vi "VCS Add Pvt Value To Ipm Buffer.vi"(0 "axis in":cluster{"keyHandle":u32, "nodeId":u16}={"keyHandle"=0, "nodeId"=1}, 7 "PVT value":T1, 11 "error in (no error)":errorcluster) -> (4 "axis out":cluster{"keyHandle":u32, "nodeId":u16}={"keyHandle"=0, "nodeId"=1}, 15 "error out":errorcluster)   [LabVIEW 2019, in "maxonEPOS.lvlib"]
doc: "The function <B>VCS_AddPvtValueToIpmBuffer</B> adds a new PVT reference point to the device."
uses:
  Examples/maxonEPOS.lvlib
  Resources/EposCmd.dll
  Resources/EposCmd64.dll
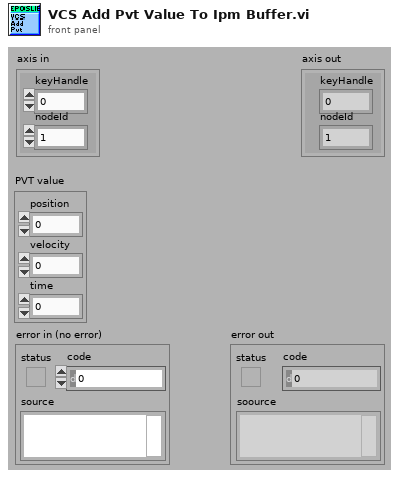
[diagram p1: front panel]
types:
  T1 = cluster{"position":i32, "velocity":i32, "time":u8}
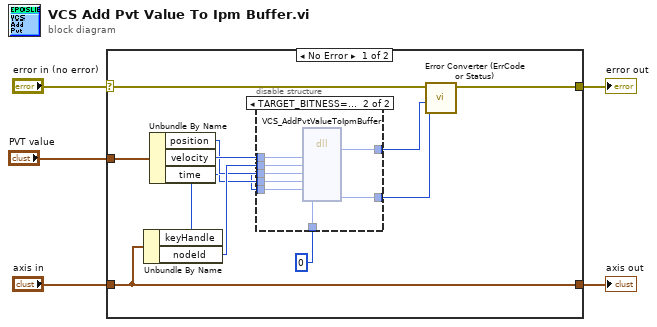
[diagram p0: block diagram]
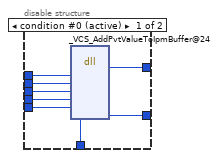
[diagram p2: hidden frame]
diagram:
  n1 = case shown="No Error" "error in (no error)" {
    selector: "error in (no error)" -> [w15 w34]
    tunnel: "axis in" -> [w17 w35]
    tunnel: [w17 w35] -> w4
    tunnel: [w16 w34] -> w3
    tunnel: "PVT value" -> [w9 _]
    frame No Error {
      n2 = Unbundle By Name(w17) -> ("keyHandle"=w11:u32, "nodeId"=w12:u16)
      n3 = Unbundle By Name(w9) -> ("position"=w8:i32, "velocity"=w7:i32, "time"=w6:u8)
      n4 = disable-structure shown="TARGET_BITNESS==64" {
        disable-tunnel: [w25 w33] -> w14
        disable-tunnel: [w24 w32] -> w13
        disable-tunnel: w12 -> [w23 w31]
        disable-tunnel: w11 -> [w22 w30]
        disable-tunnel: u32 0 ("pErrorCode") -> [w21 w29]
        disable-tunnel: w8 -> [w20 w28]
        disable-tunnel: w7 -> [w19 w27]
        disable-tunnel: w6 -> [w18 w26]
        frame condition #0 (active) {
          n5 = dll-call lib="C:/workspace/project/scancon/sw/SSI_Tool/InstrumentsInterfaces/Motordriver/maxon EPOS/Resources/EposCmd.*" fn="_VCS_AddPvtValueToIpmBuffer@24"("KeyHandle"=w22, "NodeId"=w23, "Position"=w20, "Velocity"=w19, "Time"=w18, "pErrorCode"=w21) -> (w25:i32, "pErrorCode"=w24:u32)  [unwired: 8 in, 2 out]
        }
        frame condition #1 {
          n6 = dll-call lib="C:/Sources/LabView/maxon EPOS/Resources/EposCmd64.*" fn="VCS_AddPvtValueToIpmBuffer" ("EposCmd.dll:_VCS_AddPvtValueToIpmBuffer@24")("KeyHandle"=w30, "NodeId"=w31, "Position"=w28, "Velocity"=w27, "Time"=w26, "pErrorCode"=w29) -> ("Rückgabetyp"=w33:i32, "pErrorCode"=w32:u32)  [unwired: 8 in, 2 out]
        }
      }
      n7 = call "Error Converter (ErrCode or Status).vi"("error code"=w13, "return type"=w14, "error in (no error)"=w15) -> ("error out"=w16:errorcluster)  [unwired: 7 in]
    }
    frame Error {
    }
  }
  "error out" <- w3
  "axis out" <- w4
